vi "Blink_1.vi"() -> ()   [LabVIEW 2013]
uses:
  <vilib>/LabVIEW Interface for Arduino/Type Defs/Board Type.ctl
  <vilib>/LabVIEW Interface for Arduino/Type Defs/Pin Mode.ctl
  <vilib>/LabVIEW Interface for Arduino/LabVIEW Interface for Arduino.lvlib
panel:
  out "Boolean":bool
  in  "millisecond multiple":u32(slide) scale=0.0..1000.0
  in  "stop":bool
  in  "Pin Mode (Input)":T1
  in  "Digital I/O Pin":u8(slide) scale=0.0..13.0
  in  "Board Type (Uno)":T2
  in  "VISA resource":refnum<visa-resource-name>
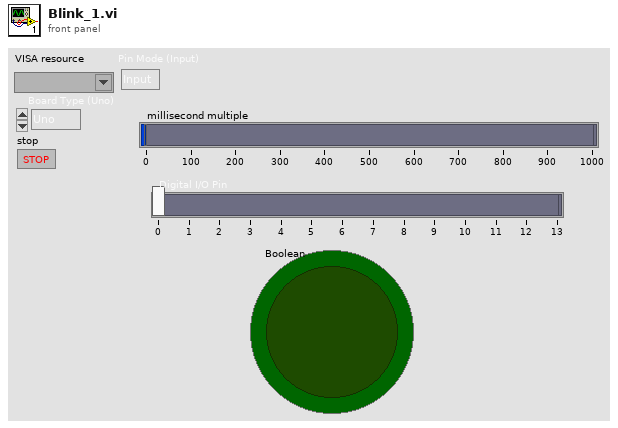
[diagram p1: front panel]
types:
  T1 = typedef "LabVIEW Interface for Arduino.lvlib/Pin Mode.ctl" = enum8{"Input", "Output"}
  T2 = typedef "LabVIEW Interface for Arduino.lvlib/Board Type.ctl" = enum16{"Uno", "Dimuelanove w/Atmega 328", "Mega 2560"}
  T3 = typedef "LabVIEW Interface for Arduino.lvlib/Arduino Resource.ctl" = cluster{"VISA resource":refnum<visa-resource-name>, "Board Type":T2, "Connection Type":enum8{"USB / Serial"}, "Bytes Per Packet (15)":u8}
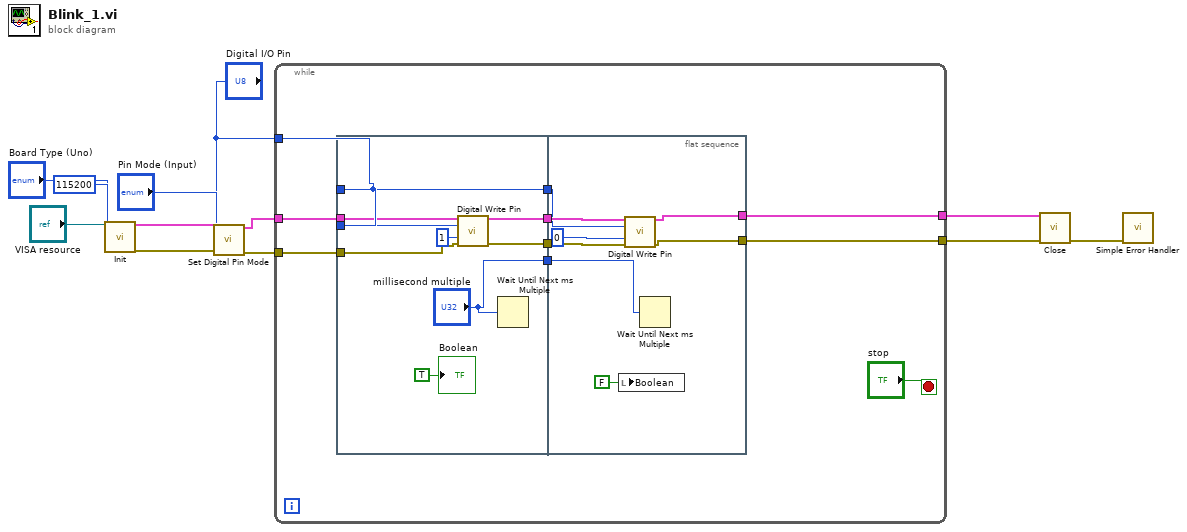
[diagram p0: block diagram]
diagram:
  n1 = call <vilib>:"Init.vi"("VISA resource"="VISA resource", "Baud Rate (115200)"=u32 115200, "Board Type (Uno)"="Board Type (Uno)") -> ("Arduino Resource"=w9:T3, "error out"=w7:errorcluster)  [unwired: 15 in]
  n2 = call <vilib>:"Set Digital Pin Mode.vi"("Arduino Resource"=w9, "Digital I/O Pin"="Digital I/O Pin", "Pin Mode (Input)"="Pin Mode (Input)", "error in"=w7) -> ("Arduino Resource"=w6:T3, "error out"=w5:errorcluster)  [unwired: 10 in]
  n3 = while {
    tunnel: w6 -> [w21]
    tunnel: w5 -> [w20]
    tunnel: "Digital I/O Pin" -> [w17]
    tunnel: [w14] -> w3
    tunnel: [w13] -> w2
    stop <- "stop" stop-if-true
    n4 = flat-sequence {
      tunnel: w21 -> [w31]
      tunnel: w20 -> [w30]
      tunnel: w17 -> [w29]
      tunnel: [w27] -> w19
      tunnel: [w26] -> w18
      tunnel: w17 -> [w25]
      tunnel: [w25] -> w16
      tunnel: ["millisecond multiple"] -> w15
      tunnel: w19 -> [w39]
      tunnel: w18 -> [w38]
      tunnel: w16 -> [w37]
      tunnel: w15 -> [w35]
      tunnel: [w33] -> w14
      tunnel: [w32] -> w13
      frame #0 {
        n5 = call <vilib>:"Digital Write Pin.vi"("Arduino Resource"=w31, "Digital I/O Pin (0)"=w29, "Value (0)"=u8 1, "error in"=w30) -> ("Arduino Resource"=w27:T3, "error out"=w26:errorcluster)  [unwired: 10 in]
        n6 = Wait Until Next ms Multiple(millisecond multiple="millisecond multiple") -> ()  [unwired: 1 out]
        "Boolean" <- TRUE ("Boolean")
      }
      frame #1 {
        n7 = local write "Boolean"(FALSE ("Boolean")) -> ()
        n8 = call <vilib>:"Digital Write Pin.vi"("Arduino Resource"=w39, "Digital I/O Pin (0)"=w37, "Value (0)"=u8 0, "error in"=w38) -> ("Arduino Resource"=w33:T3, "error out"=w32:errorcluster)  [unwired: 10 in]
        n9 = Wait Until Next ms Multiple(millisecond multiple=w35) -> ()  [unwired: 1 out]
      }
    }
  }
  n10 = call <vilib>:"Close.vi"("Arduino Resource"=w3, "error in"=w2) -> ("error out"=w1:errorcluster)  [unwired: 13 in]
  n11 = call <vilib>:"Simple Error Handler.vi"("error in (no error)"=w1) -> ()  [unwired: 4 in, 5 out]
